vi "from string.vi"(8 "error in":errorcluster, 9 "data":string, 10 "version":string, 11 "Profibus Module configuration in":refnum<class "Profibus Module configuration.lvclass">) -> (0 "error out":errorcluster, 3 "Profibus Module configuration out":refnum<class "Profibus Module configuration.lvclass">)   [LabVIEW 2013, in "Profibus Module configuration.lvclass"]
doc: "Provides an interface for loading a module configuration from a file or other serialized data source. It is recommended that all children of this class store data in two sets--data required for its own initialization, and any data required for parent initialization--and that each implementation uses the <b>Call Parent Method</b> primitive to de-serialize parent information. As a result, it is expected that every module configuration class calls <b>component configuration.lvclass:From String.vi</b>."
uses:
  Profibus Module configuration.lvclass
  <vilib>/NI/Tag Bus Module Framework/module configuration/TBM module configuration.lvclass
  Profibus Module configuration.lvclass/Profibus Module configuration.ctl
  channel/Profibus channel.lvclass
  <vilib>/NI/Tag Bus Module Framework/root configuration/TBM configuration.lvclass
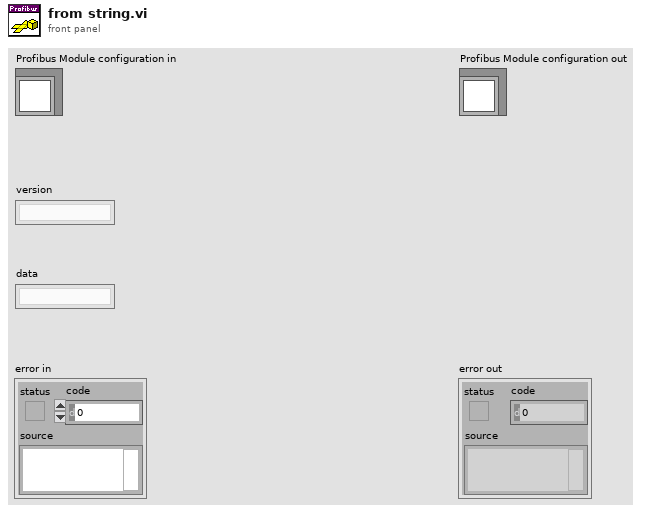
[diagram p1: front panel]
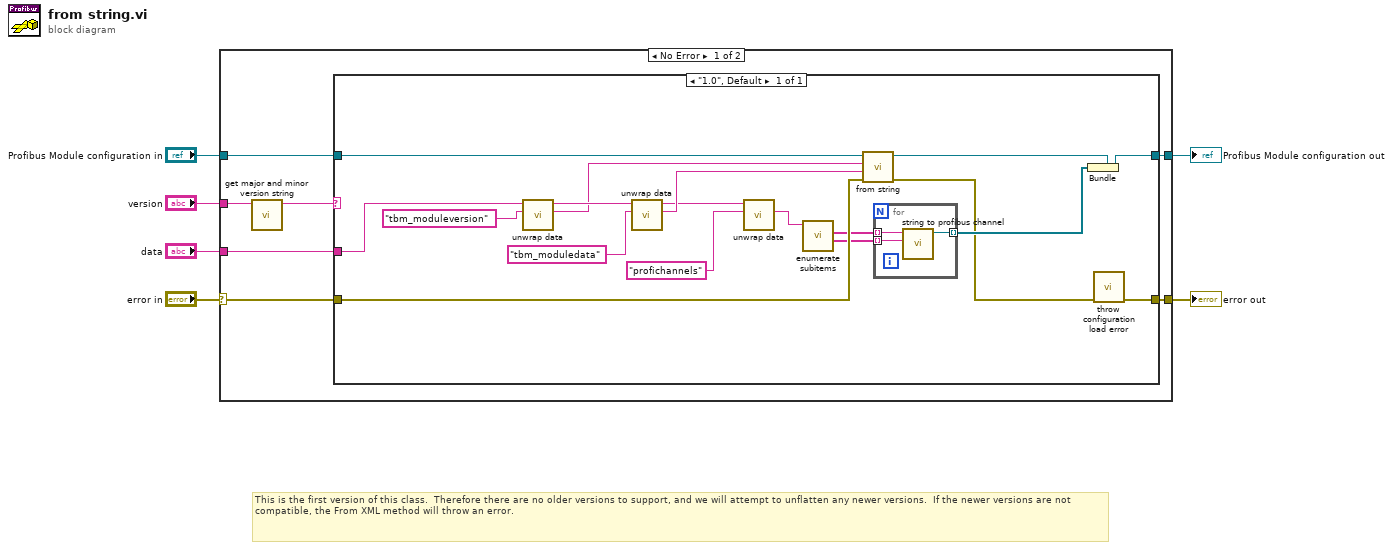
[diagram p0: block diagram]
diagram:
  # "This is the first version of this class.  Therefore there are no older versions to support, and we will attempt to unflatten any newer versions.  If the newer versions are not compatible, the From XML method will throw an error."
  n1 = case shown="No Error" "error in" {
    selector: "error in" -> [w7 w36]
    tunnel: "data" -> [w13 _]
    tunnel: "Profibus Module configuration in" -> [w12 w35]
    tunnel: [w11 w35] -> w5
    tunnel: [w10 w36] -> w4
    tunnel: "version" -> [w9 _]
    frame No Error {
      n2 = call <vilib>:"get major and minor version string.vi"("full version"=w9) -> ("major.minor version"=w8:string)  [unwired: 10 in]
      n3 = case shown="\"1.0\", Default" w8 {
        tunnel: w13 -> [w27]
        tunnel: w7 -> [w26]
        tunnel: w12 -> [w31]
        tunnel: [w21] -> w11
        tunnel: [w29] -> w10
        frame "1.0", Default {
          n4 = call <vilib>:"unwrap data.vi"("identifier"="tbm_moduleversion" ("additional identifier"), "data to unwrap"=w27) -> ("unwrapped data"=w22:string, "remaining string"=w28:string)  [unwired: 8 in]
          n5 = call <vilib>:"unwrap data.vi"("identifier"="tbm_moduledata" ("additional identifier"), "data to unwrap"=w28) -> ("unwrapped data"=w24:string, "remaining string"=w20:string)  [unwired: 8 in]
          n6 = call <vilib>:"unwrap data.vi"("identifier"="profichannels" ("additional identifier"), "data to unwrap"=w20) -> ("unwrapped data"=w18:string)  [unwired: 8 in, 1 out]
          n7 = call <vilib>:"enumerate subitems.vi"("data to enumerate"=w18) -> ("associated data"=w16:string[], "discovered subitems"=w17:string[])  [unwired: 8 in, 1 out]
          n8 = call-parent "from string.vi"("error in"=w26, "data"=w24, "version"=w22, "module configuration in"=w31) -> ("error out"=w14:errorcluster, "module configuration out"=w30:refnum<class "Profibus Module configuration.lvclass">)  [unwired: 6 in]
          n9 = for {
            tunnel: w17 -> [w34] mode=indexing
            tunnel: w16 -> [w33] mode=indexing
            tunnel: [w32] -> w15 mode=indexing
            n10 = call "string to profibus channel.vi"("channel data"=w33, "identifier"=w34) -> ("Profibus channel"=w32:refnum<class "Profibus channel.lvclass">)  [unwired: 9 in]
          }
          n11 = Bundle(cluster=w30, w15) -> (w21:refnum<class "Profibus Module configuration.lvclass">)
          n12 = call <vilib>:"throw configuration load error.vi"("error in"=w14) -> ("error out"=w29:errorcluster)  [unwired: 10 in]
        }
      }
    }
    frame Error {
    }
  }
  "error out" <- w4
  "Profibus Module configuration out" <- w5
